vi "8b.vi"() -> ()   [LabVIEW 2015]
panel:
  out "XY Graph 3":cluster{dbl[], dbl[]}(graph)
  out "XY Graph 2":cluster{dbl[], dbl[]}(graph)
  out "XY Graph":cluster{dbl[], dbl[]}(graph)
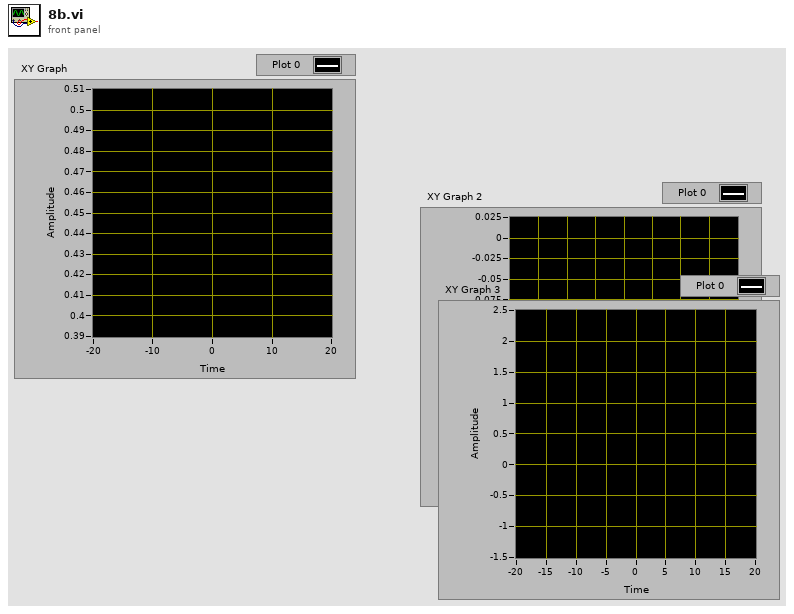
[diagram p1: front panel]
types:
  T1 = enum16{"open", "replace", "create", "open or create", "replace or create", "replace or create with confirmation"}
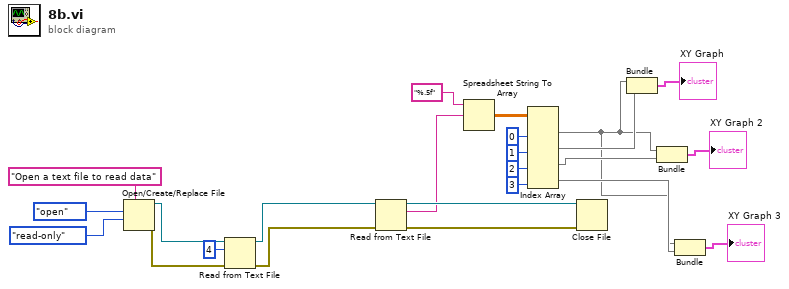
[diagram p0: block diagram]
diagram:
  n1 = Open/Create/Replace File(prompt="Open a text file to read data", operation (0:open)=T1."open", access (0:read/write)=enum16{"read/write", "read-only", "write-only"}."read-only") -> (refnum out=w12:refnum<file>, error out=w11:errorcluster)  [unwired: 3 in, 1 out]
  n2 = Read from Text File(file (use dialog)=w12, count=4, error in=w11) -> (refnum out=w10:refnum<file>, error out=w9:errorcluster)  [unwired: 1 in, 2 out]
  n3 = Read from Text File(file (use dialog)=w10, error in=w9) -> (refnum out=w24:refnum<file>, text=w18:string, error out=w23:errorcluster)  [unwired: 2 in, 1 out]
  n4 = Spreadsheet String To Array(format string="%.5f", spreadsheet string=w18) -> (array=w19:dbl[][])  [unwired: 2 in]
  n5 = Index Array(array=w19, index (col) #1=0 ("disabled index (col)"), index (col) #2=1 ("index (col)"), index (col) #3=2 ("index (col)"), index (col) #4=3 ("index (col)")) -> (element #1=w1:dbl[], element #2=w7:dbl[], element #3=w3:dbl[], element #4=w2:dbl[])  [unwired: 4 in]
  n6 = Close File(refnum=w24, error in=w23) -> ()  [unwired: 2 out]
  n7 = Bundle(w1, w7) -> (→"XY Graph":cluster{dbl[], dbl[]})  [unwired: 1 in]
  n8 = Bundle(w1, w3) -> (→"XY Graph 2":cluster{dbl[], dbl[]})  [unwired: 1 in]
  n9 = Bundle(w1, w2) -> (→"XY Graph 3":cluster{dbl[], dbl[]})  [unwired: 1 in]
